vi "Format JSON Array Text.vi"(6 "Pretty Print?":bool, 8 "error in (no error)":errorcluster, 10 "Array of JSON Text":string[](array[string])) -> (0 "error out":errorcluster, 3 "<JSON>":string)   [LabVIEW 2020, in "JSONtext.lvlib"]
uses:
  <vilib>/JDP Science/JSONtext/JSONtext.lvlib
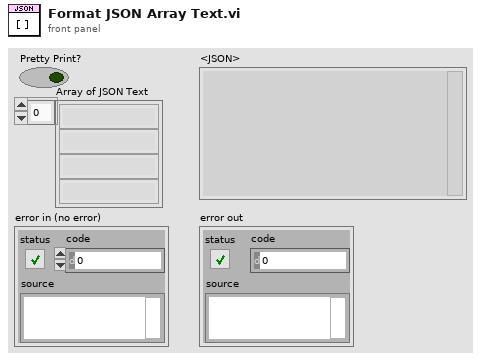
[diagram p1: front panel]
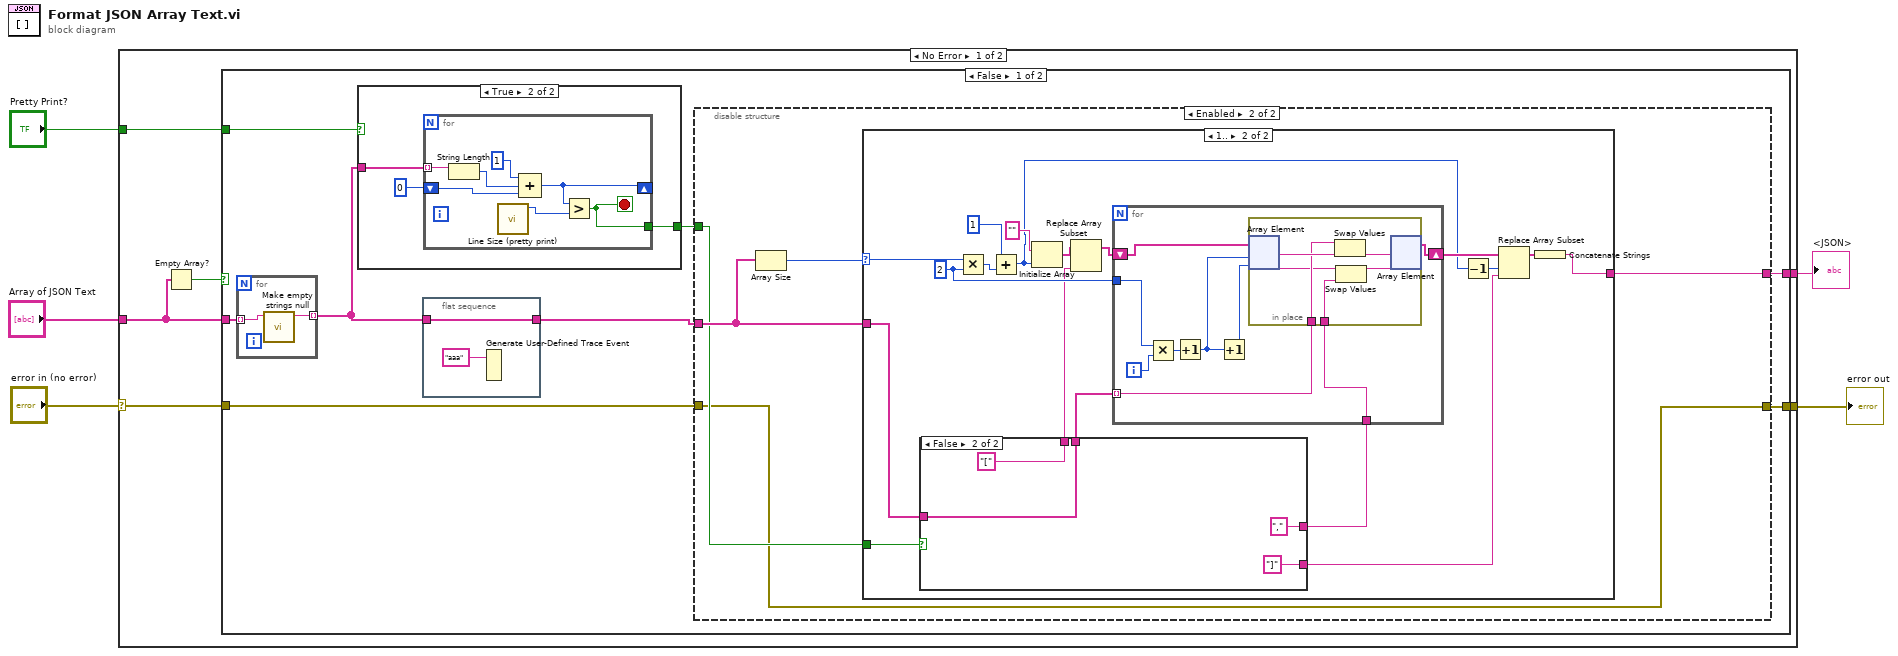
[diagram p0: block diagram]
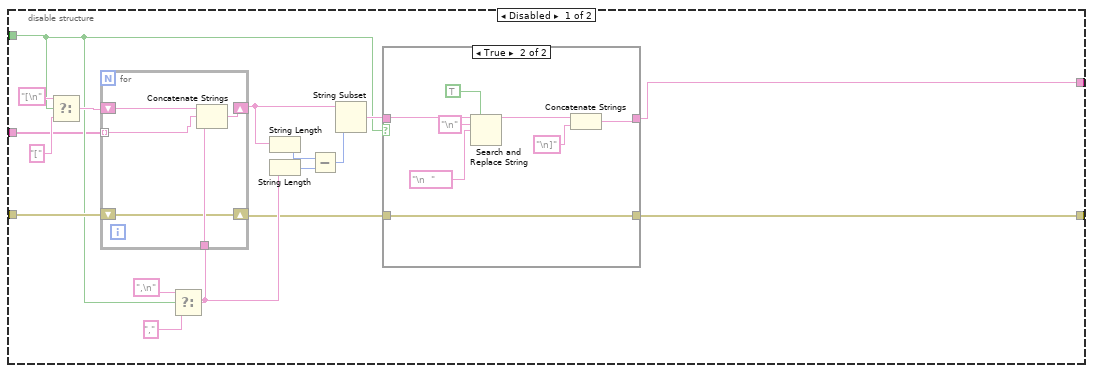
[diagram p2: hidden frame]
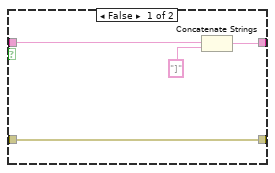
[diagram p3: hidden frame]
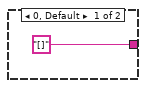
[diagram p4: hidden frame]
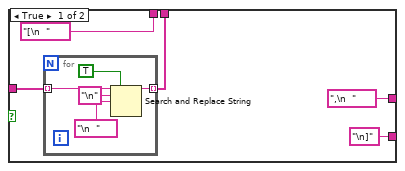
[diagram p5: hidden frame]
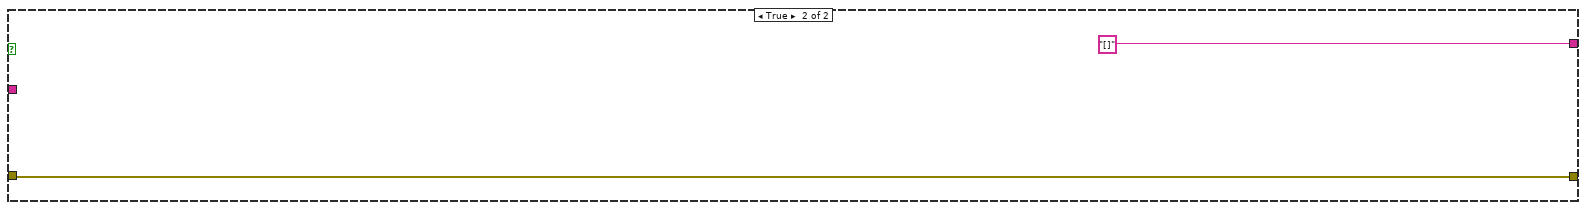
[diagram p7: hidden frame]
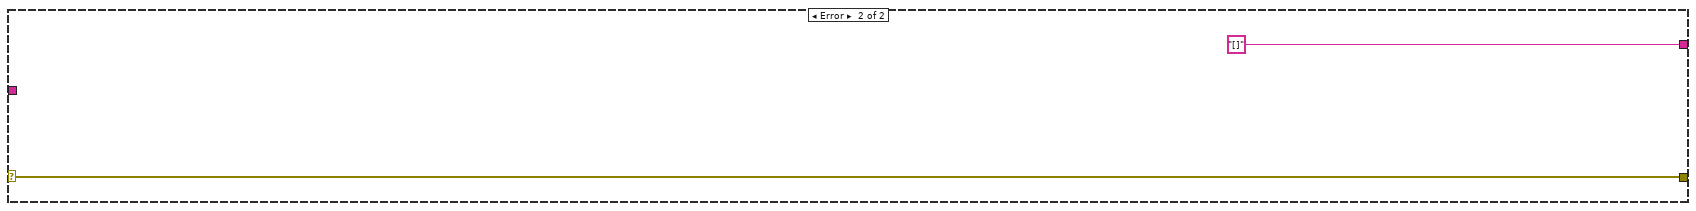
[diagram p8: hidden frame]
diagram:
  n1 = case shown="No Error" "error in (no error)" {
    selector: "error in (no error)" -> [w10 w124]
    tunnel: [w11 "[]" ("t")] -> w5
    tunnel: "Pretty Print?" -> [w9 _]
    tunnel: "Array of JSON Text" -> [w7 _]
    tunnel: [w8 w124] -> w1
    frame No Error {
      n2 = Empty Array?(array=w7) -> (empty?=w6:bool)
      n3 = case shown="False" w6 {
        tunnel: [w18 "[]" ("t")] -> w11
        tunnel: w10 -> [w19 w121]
        tunnel: w9 -> [w17 _]
        tunnel: [w15 w121] -> w8
        tunnel: w7 -> [w14 _]
        frame False {
          n4 = for {
            tunnel: w14 -> [w120] mode=indexing
            tunnel: [w119] -> w16 mode=indexing
            n5 = call <vilib>:"Make empty strings null.vi"("JSON Input"=w120) -> ("<JSON>"=w119:string)  [unwired: 10 in]
          }
          n6 = case shown="True" w17 {
            tunnel: w16 -> [_ w111]
            tunnel: [_ w109] -> w13
            frame False {
            }
            frame True {
              n7 = for {
                tunnel: w111 -> [w118] mode=indexing
                shift-right: [w116] -> _
                shift-left: 0 -> [w117]
                tunnel: [w115] -> w109
                stop <- w115 stop-if-true
                n8 = String Length(string=w118) -> (length=w114:i32)
                n9 = call <vilib>:"Line Size (pretty print).vi"() -> ("Line Size"=w113:i32)  [unwired: 11 in]
                n10 = Compound Arithmetic op=ADD(1 ("value"), w114, w117) -> (w116:i32)
                n11 = Greater?(x=w116, y=w113) -> (0:w115:bool)
              }
            }
          }
          n12 = flat-sequence {
            tunnel: [w20] -> w12
            tunnel: w16 -> [w20]
            frame #0 {
              n13 = Generate User-Defined Trace Event(2:"aaa" ("trace string")) -> ()  [unwired: 1 in]
            }
          }
          n14 = disable-structure shown="Enabled" {
            disable-tunnel: w19 -> [w38 w56]
            disable-tunnel: [w37 w59] -> w18
            disable-tunnel: w13 -> [w25 w57]
            disable-tunnel: w12 -> [w24 w58]
            disable-tunnel: [w22 w56] -> w15
            frame Disabled {
              n15 = Select(t="[\n", s=w25, f="[") -> (s? t:f=w32:string)
              n16 = Select(t=",\n" ("string"), s=w25, f="," ("string")) -> (s? t:f=w36:string)
              n17 = for {
                tunnel: w24 -> [w52] mode=indexing
                shift-right: [w55] -> w28
                shift-left: w32 -> [w54]
                shift-right: [w51] -> w23
                shift-left: w38 -> [w51]
                tunnel: w36 -> [w53]
                n18 = Concatenate Strings(w54, w52, w53) -> (w55:string)
              }
              n19 = String Length(string=w28) -> (length=w29:i32)
              n20 = String Length(string=w36) -> (length=w30:i32)
              n21 = Subtract(x=w29, y=w30) -> (x-y=w31:i32)
              n22 = String Subset(string=w28, length (rest)=w31) -> (substring=w33:string)  [unwired: 1 in]
              n23 = case shown="True" w25 {
                tunnel: w33 -> [w40 w46]
                tunnel: [w41 w47] -> w37
                tunnel: w23 -> [w39 w43]
                tunnel: [w39 w43] -> w22
                frame False {
                  n24 = Concatenate Strings(w40, "]" ("substring (\"\")")) -> (w41:string)
                }
                frame True {
                  n25 = Search and Replace String(replace all?=TRUE ("replace all? (F)"), input string=w46, search string="\n", replace string="\n  " ("search string")) -> (result string=w48:string)  [unwired: 4 in, 3 out]
                  n26 = Concatenate Strings(w48, "\n]" ("search string")) -> (w47:string)
                }
              }
            }
            frame Enabled {
              n27 = Array Size(array=w58) -> (size(s)=w60:i32)
              n28 = case shown="1.." w60 {
                selector: w60 -> [_ w65]
                tunnel: ["[]" w63] -> w59
                tunnel: w58 -> [_ w64]
                tunnel: w57 -> [_ w62]
                frame 0, Default {
                }
                frame 1.. {
                  w77 = 2 ("y")
                  n29 = case shown="False" w62 {
                    tunnel: [",\n  " ("new element/subarray") "," ("new element/subarray")] -> w76
                    tunnel: ["\n]" ("new element/subarray") "]" ("new element/subarray")] -> w68
                    tunnel: w64 -> [w82 w91]
                    tunnel: [w81 w91] -> w67
                    tunnel: ["[\n  " ("new element/subarray") "[" ("new element/subarray")] -> w66
                    frame True {
                      n30 = for {
                        tunnel: w82 -> [w86] mode=indexing
                        tunnel: [w85] -> w81 mode=indexing
                        n31 = Search and Replace String(replace all?=TRUE ("replace all? (F)"), input string=w86, search string="\n", replace string="\n  " ("search string")) -> (result string=w85:string)  [unwired: 4 in, 3 out]
                      }
                    }
                    frame False {
                    }
                  }
                  n32 = Multiply(x=w65, y=w77) -> (x*y=w79:i32)
                  n33 = Add(x=1, y=w79) -> (x+y=w69:i32)
                  n34 = Initialize Array("", w69) -> (w73:string[])
                  n35 = Replace Array Subset(array=w73, new element=w66) -> (w74:string[])  [unwired: 1 in]
                  n36 = for {
                    tunnel: w67 -> [w97] mode=indexing
                    shift-right: [w94] -> w72
                    shift-left: w74 -> [w99]
                    tunnel: w77 -> [w101]
                    tunnel: w76 -> [w96]
                    i -> [w102]
                    n37 = Multiply(x=w101, y=w102) -> (x*y=w100:i32)
                    n38 = Increment(x=w100) -> (x+1=w98:i32)
                    n39 = Increment(x=w98) -> (x+1=w95:i32)
                    n40 = in-place {
                      in-place-border: w97 -> [w106]
                      in-place-border: w96 -> [w105]
                      n41 = in-place-array #1(w99, w98, w95) -> (w108:string, w104:string)
                      n42 = Swap Values(12:w106, 14:w108) -> (3:w107:string)  [unwired: 1 in, 1 out]
                      n43 = Swap Values(12:w104, 14:w105) -> (1:w103:string)  [unwired: 1 in, 1 out]
                      n44 = in-place-array #1(w107, w103) -> (w94:string[])  [unwired: 2 out]
                    }
                  }
                  n45 = Decrement(x=w69) -> (x-1=w70:i32)
                  n46 = Replace Array Subset(array=w72, new element=w68, index=w70) -> (w71:string[])
                  n47 = Concatenate Strings(w71) -> (w63:string)
                }
              }
            }
          }
        }
        frame True {
        }
      }
    }
    frame Error {
    }
  }
  "<JSON>" <- w5
  "error out" <- w1
